vi "19052 PreSet_AFTER_FAIL.vi"(8 "error in (no error)":errorcluster, 10 "Operation":u16(ring) items=["STOP", "CONTinue", "RESTart"], 11 "VISA resource in":refnum<visa-resource-name>) -> (0 "error out":errorcluster, 2 "output command":string, 3 "VISA resource out":refnum<visa-resource-name>)   [LabVIEW 2015]
doc: "This VI writes to the instrument the AFTER FAIL posible values."
panel:
  # "PreSet AFTER FAIL"
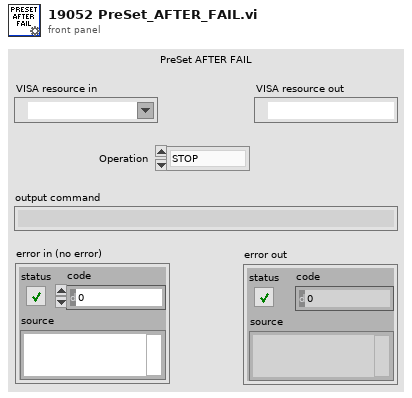
[diagram p1: front panel]
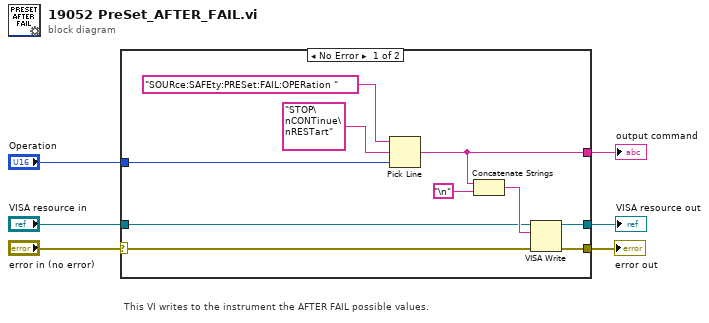
[diagram p0: block diagram]
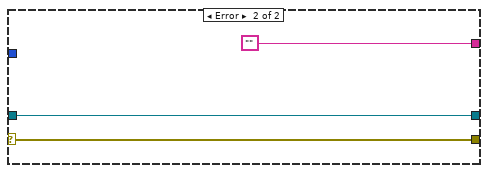
[diagram p2: hidden frame]
diagram:
  # "This VI writes to the instrument the AFTER FAIL possible values."
  n1 = case shown="No Error" "error in (no error)" {
    selector: "error in (no error)" -> [w15 w19]
    tunnel: [w16 w19] -> w6
    tunnel: "Operation" -> [w10 _]
    tunnel: "VISA resource in" -> [w9 w18]
    tunnel: [w8 ""] -> w2
    tunnel: [w7 w18] -> w1
    frame No Error {
      n2 = Pick Line(string ("")="SOURce:SAFEty:PRESet:FAIL:OPERation ", multi-line string="STOP\nCONTinue\nRESTart", line index=w10) -> (output string=w8:string)
      n3 = Concatenate Strings(w8, "\n") -> (w12:string)
      n4 = VISA Write(VISA resource name=w9, write buffer=w12, error in (no error)=w15) -> (VISA resource name out=w7:refnum<visa-resource-name>, error out=w16:errorcluster)  [unwired: 1 out]
    }
    frame Error {
    }
  }
  "error out" <- w6
  "VISA resource out" <- w1
  "output command" <- w2
